vi "centroid_subvi.vi"(0 "Refnum in":T1) -> (1 "Refnum out":T1, 2 "Centroid":cluster{"X Centroid":sgl, "Y Centroid":sgl} {"Y Centroid" format="%.2f"; "X Centroid" format="%.2f"})   [LabVIEW 2020]
uses:
  <vilib>/vision/Image Controls.llb/IMAQ Image.ctl
  <vilib>/vision/NI_Vision_Development_Module.lvlib
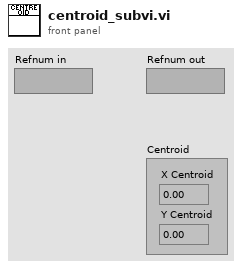
[diagram p1: front panel]
types:
  T1 = typedef "IMAQ Image.ctl" = refnum<image>
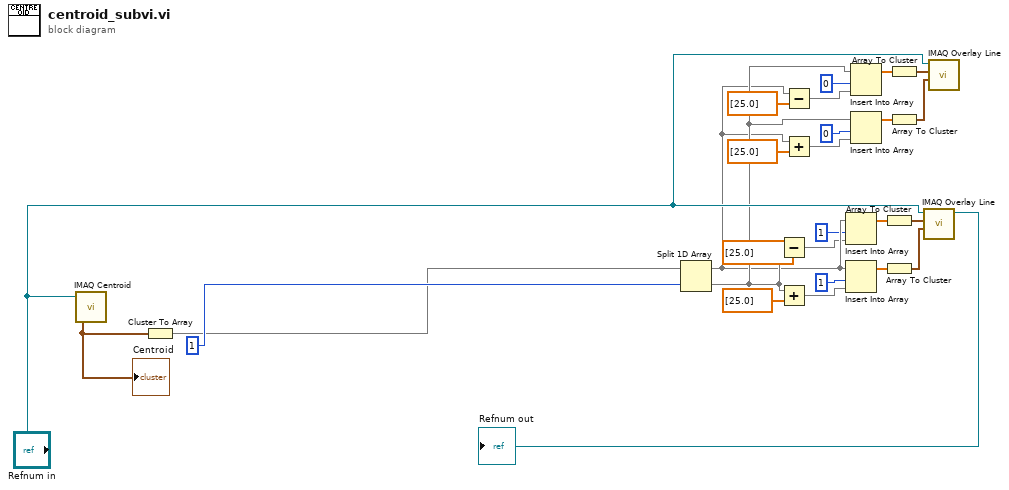
[diagram p0: block diagram]
diagram:
  n1 = call "IMAQ Centroid"("Image"="Refnum in") -> ("Centroid"=w1:cluster{"X Centroid":sgl, "Y Centroid":sgl})  [unwired: 3 in, 1 out]
  "Centroid" <- w1
  n2 = Cluster To Array(cluster=w1) -> (array=w2:sgl[])
  n3 = Split 1D Array(array=w2, index=1) -> (first subarray=w25:sgl[], second subarray=w26:sgl[])
  n4 = Subtract(x=w26, y=sgl[] [25.0]) -> (x-y=w9:sgl[])
  n5 = Add(x=w26, y=sgl[] [25.0]) -> (x+y=w6:sgl[])
  n6 = Subtract(x=w25, y=sgl[] [25.0]) -> (x-y=w20:sgl[])
  n7 = Add(x=w25, y=sgl[] [25.0]) -> (x+y=w17:sgl[])
  n8 = Insert Into Array(array=w25, index=1, new element=w9) -> (w10:sgl[])
  n9 = Insert Into Array(array=w25, index=1, new element=w6) -> (w12:sgl[])
  n10 = Insert Into Array(array=w26, index=0, new element=w20) -> (w21:sgl[])
  n11 = Insert Into Array(array=w26, index=0, new element=w17) -> (w23:sgl[])
  n12 = Array To Cluster(array=w10) -> (cluster=w11:cluster{"[0]":sgl, "[1]":sgl})
  n13 = Array To Cluster(array=w12) -> (cluster=w13:cluster{"[0]":sgl, "[1]":sgl})
  n14 = Array To Cluster(array=w21) -> (cluster=w22:cluster{"[0]":sgl, "[1]":sgl})
  n15 = Array To Cluster(array=w23) -> (cluster=w24:cluster{"[0]":sgl, "[1]":sgl})
  n16 = call "IMAQ Overlay Line"("End Point"=w13, "Start Point"=w11, "Image"="Refnum in") -> ("Image Out"=→"Refnum out":T1)  [unwired: 7 in, 1 out]
  n17 = call "IMAQ Overlay Line"("End Point"=w24, "Start Point"=w22, "Image"="Refnum in") -> ()  [unwired: 7 in, 2 out]
